vi "Load DBC.vi"(8 "error in":errorcluster, 9 "Cluster Name":string, 10 "DBC File":string, 11 "DBCCommunication in":refnum<class "DBC Communication.lvclass">) -> (0 "error out":errorcluster, 3 "DBCCommunication out":refnum<class "DBC Communication.lvclass">)   [LabVIEW 2024, in "DBC Communication.lvclass"]
uses:
  DBC Communication.lvclass
  DBC Communication.lvclass/DBC Communication.ctl
  <resource>/objmgr/xnet.rc
  <vilib>/xnet/xnet.llb/XNET Create Session (Conversion).vi
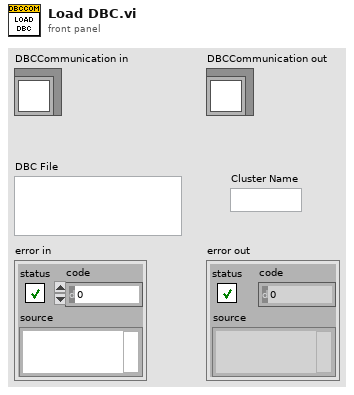
[diagram p1: front panel]
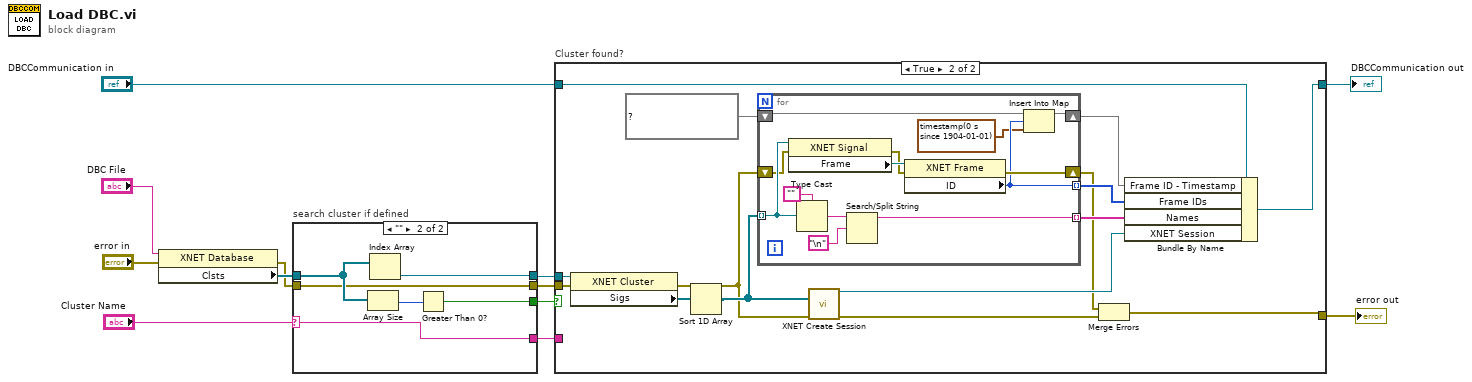
[diagram p0: block diagram]
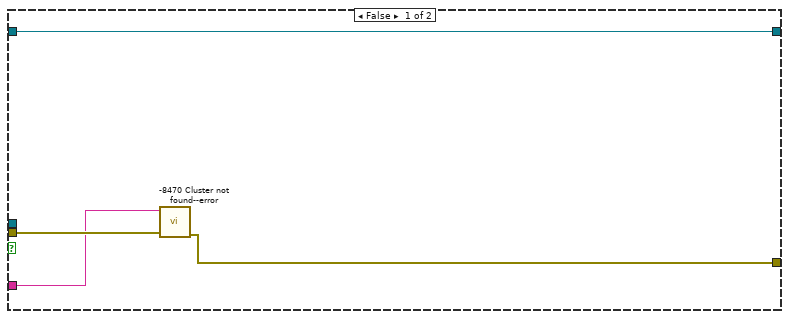
[diagram p2: hidden frame]
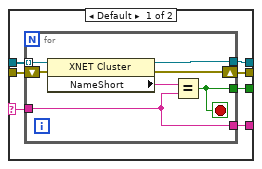
[diagram p3: hidden frame]
diagram:
  n1 = property class="XNET Database"(reference="DBC File", error in="error in") -> (error out=w6:errorcluster, "Clsts"=w7:refnum<k21>[])  [unwired: 1 out]
  n2 = case "search cluster if defined" shown="\"\"" "Cluster Name" {
    selector: "Cluster Name" -> [w18 w28]
    tunnel: w7 -> [w19 w31]
    tunnel: [w17 w32] -> w4
    tunnel: [w16 w29] -> w2
    tunnel: [w15 w28] -> w1
    tunnel: w6 -> [w14 w27]
    tunnel: [w13 w27] -> w5
    frame Default {
      n3 = for {
        tunnel: [w26] -> w17
        tunnel: w19 -> [w25] mode=indexing
        tunnel: w18 -> [w22]
        tunnel: [w23] -> w16
        tunnel: [w22] -> w15
        shift-right: [w20] -> w13
        shift-left: w14 -> [w21]
        stop <- w23 stop-if-true
        n4 = property class="XNET Cluster"(reference=w25, error in=w21) -> (reference out=w26:refnum<k21>, error out=w20:errorcluster, "NameShort"=w24:string)
        n5 = Equal?(x=w24, y=w22) -> (x = y?=w23:bool)
      }
    }
    frame "" {
      n6 = Array Size(array=w31) -> (size(s)=w30:i32)
      n7 = Index Array(array=w31) -> (element=w32:refnum<k21>)  [unwired: 1 in]
      n8 = Greater Than 0?(x=w30) -> (x > 0?=w29:bool)
    }
  }
  n9 = case "Cluster found?" shown="True" w2 {
    tunnel: "DBCCommunication in" -> [w33 w48]
    tunnel: [w33 w46] -> w9
    tunnel: [w34 w37] -> w8
    tunnel: w5 -> [w36 w44]
    tunnel: w4 -> [_ w43]
    tunnel: w1 -> [w35 _]
    frame False {
      n10 = call "-8470 Cluster not found--error.vi"("error in"=w36, "Cluster Name"=w35) -> ("error out"=w34:errorcluster)  [unwired: 9 in]
    }
    frame True {
      n11 = property class="XNET Cluster"(reference=w43, error in=w44) -> (error out=w42:errorcluster, "Sigs"=w50:refnum<k21>[])  [unwired: 1 out]
      n12 = Sort 1D Array(array=w50) -> (sorted array=w49:refnum<k21>[])
      n13 = for {
        tunnel: w49 -> [w60] mode=indexing
        tunnel: [w62] -> w51 mode=indexing
        shift-right: [w56] -> w40
        shift-left: w42 -> [w57]
        tunnel: [w54] -> w41 mode=indexing
        shift-right: [w52] -> w39
        shift-left: map{u32, timestamp} {} ("Size: 0") -> [w55]
        n14 = property class="XNET Signal"(reference=w60, error in=w57) -> (error out=w58:errorcluster, "Frame"=w59:refnum<k21>)  [unwired: 1 out]
        n15 = Type Cast(type="", x=w60) -> (*(type *) &x=w63:string)
        n16 = Search/Split String(string=w63, search string/char (-)="\n") -> (substring before match=w62:string)  [unwired: 1 in, 2 out]
        n17 = property class="XNET Frame"(reference=w59, error in=w58) -> (error out=w56:errorcluster, "ID"=w54:u32)  [unwired: 1 out]
        n18 = Insert Into Map(map in=w55, key=w54, value=timestamp(0 s since 1904-01-01)) -> (map out=w52:map{u32, timestamp})  [unwired: 2 out]
      }
      n19 = call-poly <vilib>:"XNET Create Session.vi"("signal list"=w49, "error in (no error)"=w42) -> ("session out"=w47:refnum<k21>, "error out"=w45:errorcluster)  [unwired: 12 in]
      n20 = Merge Errors(w40, w45) -> (w37:errorcluster)
      n21 = Bundle By Name(cluster=w48, "Frame ID - Timestamp"=w39, "Frame IDs"=w41, "Names"=w51, "XNET Session"=w47) -> (w46:refnum<class "DBC Communication.lvclass">)
    }
  }
  "error out" <- w8
  "DBCCommunication out" <- w9
